vi "DAC_Xmit_order.vi"(9 "Order in":u64, 11 "FPGA VI Reference In":T1) -> (0 "error out":errorcluster, 3 "FPGA VI Reference Out":T1)   [LabVIEW 2013]
uses:
  fpga-bitfile-ref.ctl
  <vilib>/Utility/error.llb/Error Cluster From Error Code.vi
  <vilib>/rvi/errors/niLvFpgaAdjustHostInterfaceError.vi
  <vilib>/rvi/interface/nirviReadWriteControl/nirviReadWriteControl.xnode
  FPGA Bitfiles/fpga-clean1_FPGATarget_FPGAMAINlock-in_FC21E42C.lvbitx
  NiFpgaLv.dll
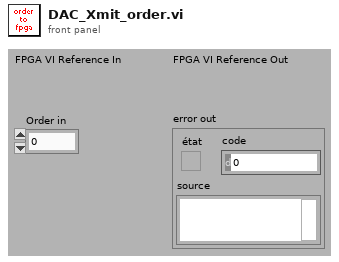
[diagram p1: front panel]
types:
  T1 = typedef "fpga-bitfile-ref.ctl" = refnum<k20>
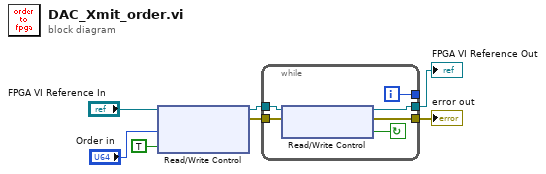
[diagram p0: block diagram]
diagram:
  n1 = xnode "Read/Write Control"("FPGA VI Reference In"="FPGA VI Reference In", "order in"="Order in", "order Xmitted"=TRUE) -> ("FPGA VI Reference Out"=w7:T1, "error out"=w6:errorcluster)  [unwired: 1 in]
  n2 = while {
    tunnel: w7 -> [w13]
    tunnel: [w12] -> w2
    tunnel: [w11] -> w1
    tunnel: w6 -> [w10]
    tunnel: [w8] -> _
    i -> [w8]
    stop <- w9 continue-if-true
    n3 = xnode "Read/Write Control"("FPGA VI Reference In"=w13, "error in"=w10) -> ("FPGA VI Reference Out"=w12:T1, "error out"=w11:errorcluster, "order Xmitted"=w9:bool)
  }
  "error out" <- w1
  "FPGA VI Reference Out" <- w2
